vi "Get SPI init FIFo elements for card.vi"(9 "Num of SPI ICs":u8=8, 11 "Card Position":T1) -> (2 "init FIFO elements":u32[](array[numeric]))   [LabVIEW 2014, in "SLSC configuration System Explorer.lvlib"]
uses:
  SLSC configuration System Explorer.lvlib
  Shared/Card Postion.ctl
  Shared/SLSC configuration Shared.lvlib
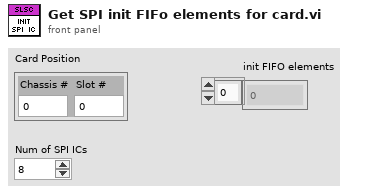
[diagram p1: front panel]
types:
  T1 = typedef "SLSC configuration Shared.lvlib/Card Postion.ctl" = cluster{"Chassis #":u8, "Slot #":u8}
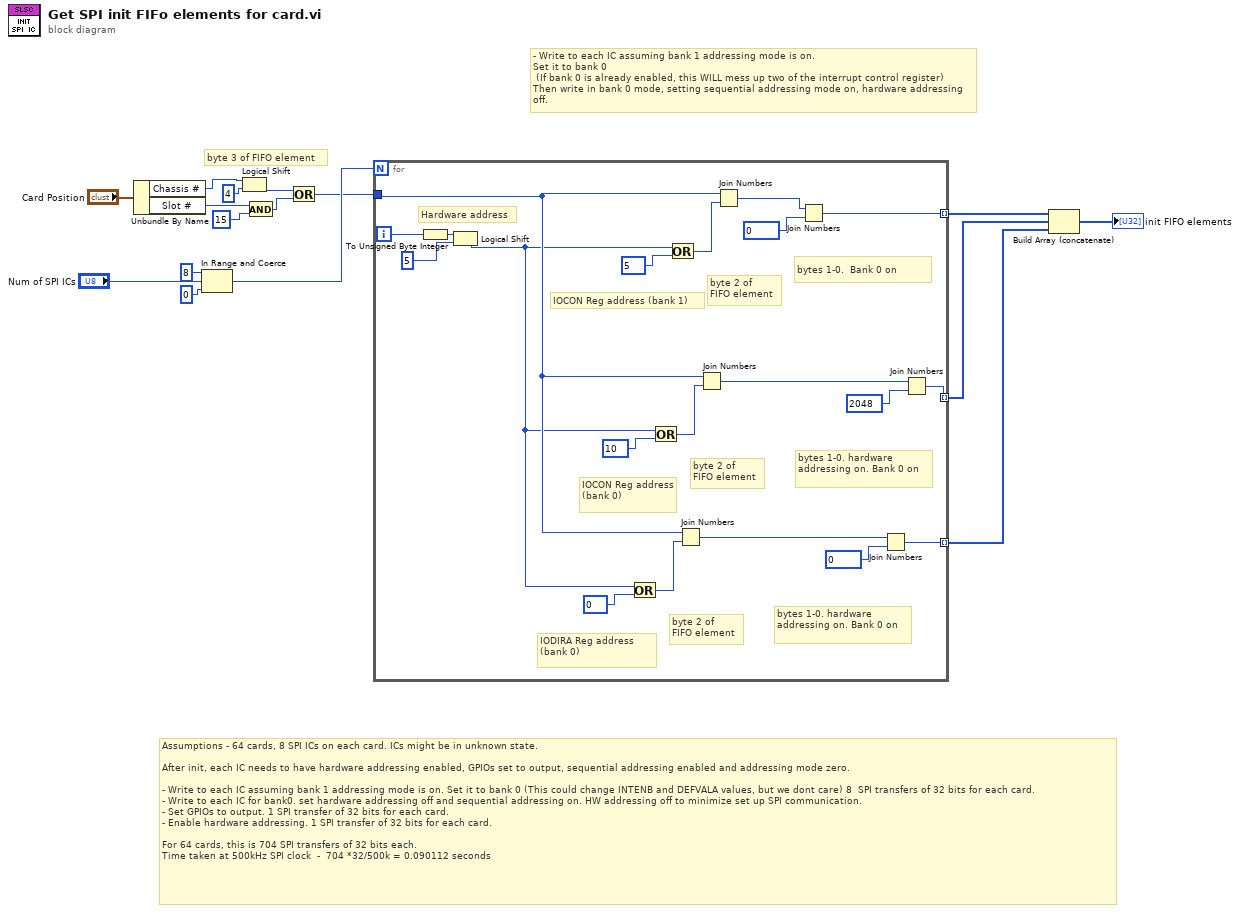
[diagram p0: block diagram]
diagram:
  # "-\tWrite to each IC assuming bank 1 addressing mode is on. \nSet it to bank 0 \n (If bank 0 is already enabled, this WILL mess up two of the interrupt control register) \nThen write in bank 0 mode, setting sequential addressing mode on, hardware addressing off."
  # "Assumptions - 64 cards, 8 SPI ICs on each card. ICs might be in unknown state.\n\nAfter init, each IC needs to have hardware addressing enabled, GPIOs set to output, sequential addressing enabled and addressing mode zero. \n\n-\tWrite to each IC assuming bank 1 addressing mode is on. Set it to bank 0 (This could change INTENB and DEFVALA values, but we dont care) 8  SPI transfers of 32 bits for each card.\n- Write to each IC for bank0. set hardware addressing off and sequential addressing on. HW addressing off to minimize set up SPI communication. \n-\tSet GPIOs to output. 1 SPI transfer of 32 bits for each card.\n-\tEnable hardware addressing. 1 SPI transfer of 32 bits for each card.\n\nFor 64 cards, this is 704 SPI transfers of 32 bits each.\nTime taken at 500kHz SPI clock  -  704 *32/500k = 0.090112 seconds"
  # "byte 3 of FIFO element"
  n1 = Unbundle By Name("Card Position") -> ("Chassis #"=w10:u8, "Slot #"=w15:u8)
  n2 = In Range and Coerce(upper limit=u8 8, x="Num of SPI ICs", lower limit=u8 0) -> (coerced(x)=w8:u8)  [unwired: 1 out]
  n3 = Logical Shift(y=w10, x=u8 4) -> (x << y=w11:u8)
  n4 = And(x=w15, y=u8 15) -> (x .and. y?=w13:u8)
  n5 = Or(x=w11, y=w13) -> (x .or. y?=w5:u8)
  n6 = for {
    N: w8 -> [_]
    tunnel: w5 -> [w19]
    tunnel: [w33] -> w4 mode=indexing
    tunnel: [w29] -> w3 mode=indexing
    tunnel: [w17] -> w2 mode=indexing
    i -> [w28]
    # "bytes 1-0. hardware addressing on. Bank 0 on"
    # "byte 2 of \nFIFO element"
    # "IODIRA Reg address (bank 0)"
    # "bytes 1-0. hardware addressing on. Bank 0 on"
    # "byte 2 of \nFIFO element"
    # "IOCON Reg address (bank 0)"
    # "bytes 1-0.  Bank 0 on"
    # "byte 2 of \nFIFO element"
    # "Hardware address"
    # "IOCON Reg address (bank 1)"
    n7 = To Unsigned Byte Integer(number=w28) -> (unsigned 8bit integer=w35:u8)
    n8 = Logical Shift(y=w35, x=u8 5) -> (x << y=w18:u8)
    n9 = Or(x=w18, y=u8 0 ("x")) -> (x .or. y?=w21:u8)
    n10 = Or(x=w18, y=u8 10 ("x")) -> (x .or. y?=w30:u8)
    n11 = Or(x=w18, y=u8 5 ("x")) -> (x .or. y?=w34:u8)
    n12 = Join Numbers(hi=w19, lo=w21) -> ((hi.lo)=w23:u16)
    n13 = Join Numbers(hi=w19, lo=w30) -> ((hi.lo)=w24:u16)
    n14 = Join Numbers(hi=w19, lo=w34) -> ((hi.lo)=w26:u16)
    n15 = Join Numbers(hi=w26, lo=u16 0 ("x")) -> ((hi.lo)=w33:u32)
    n16 = Join Numbers(hi=w23, lo=u16 0 ("x")) -> ((hi.lo)=w17:u32)
    n17 = Join Numbers(hi=w24, lo=u16 2048 ("x")) -> ((hi.lo)=w29:u32)
  }
  n18 = Build Array (concatenate)(w4, w3, w2) -> (→"init FIFO elements":u32[])
